vi "CardChannel2MuxChannel.vi"(7 "Probe Card Channels":i32=32, 8 "error in (no error)":errorcluster, 10 "Probecard Channel No.":i32=1 min=1 max=32 step=1, 11 "Switching in":refnum<class "Switching.lvclass">) -> (0 "error out":errorcluster, 1 "C1 / C2":i32=1 min=1 max=2 step=1, 2 "Mux No.:":u32(ring)=1 items=["", "", "", "", "MUX1", "MUX2"], 3 "Switching out":refnum<class "Switching.lvclass">, 4 "Channel":i32=1 min=1 max=8 step=1, 5 "Mux No. string":string)   [LabVIEW 2013, in "Switching.lvclass"]
uses:
  Switching.lvclass
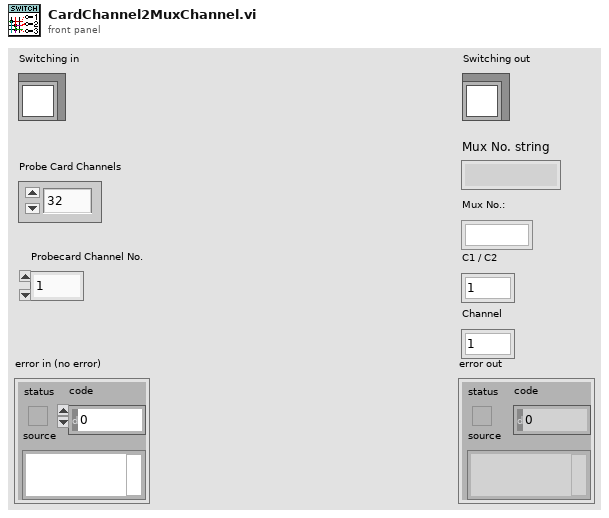
[diagram p1: front panel]
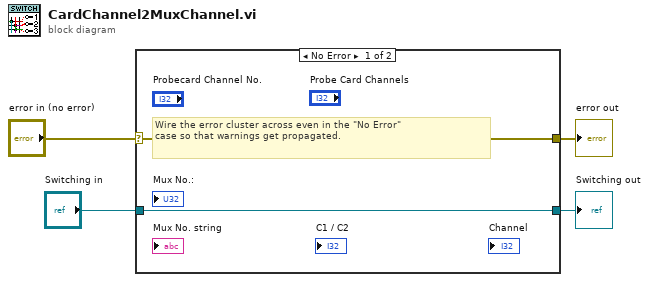
[diagram p0: block diagram]
diagram:
  n1 = case shown="No Error" "error in (no error)" {
    selector: "error in (no error)" -> [w5 w8]
    tunnel: [w5 w8] -> w3
    tunnel: [w6 w7] -> w1
    tunnel: "Switching in" -> [w6 w7]
    frame No Error {
      # "Wire the error cluster across even in the \"No Error\"\ncase so that warnings get propagated."
    }
    frame Error {
    }
  }
  "error out" <- w3
  "Switching out" <- w1
